vi "Get Processes.vi"(11 "Assembler in":refnum<class "Assembler.lvclass">) -> (2 "Processes":refnum<class "Process.lvclass">[](array[class]), 3 "Assembler out":refnum<class "Assembler.lvclass">)   [LabVIEW 2019, in "TimingDRV Engine.lvlib" / "Assembler.lvclass"]
uses:
  Assembler.lvclass
  Parent Classes/Process/Process.lvclass
  Assembler.lvclass/Assembler.ctl
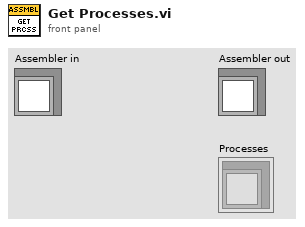
[diagram p1: front panel]
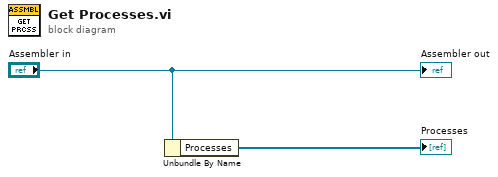
[diagram p0: block diagram]
diagram:
  n1 = Unbundle By Name("Assembler in") -> ("Processes"=→"Processes":refnum<class "Process.lvclass">[])
  "Assembler out" <- "Assembler in"
